vi "generate_list.vi"(9 "Interval":sgl, 10 "End":sgl, 11 "Start":sgl) -> (3 "Array":sgl[](array[numeric]))   [LabVIEW 2020, in "3DPC_SurfacePlot.xctl"]
uses:
  <vilib>/Native 3D Graph/xcontrol/3DPC_SurfacePlot.xctl
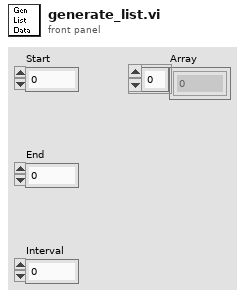
[diagram p1: front panel]
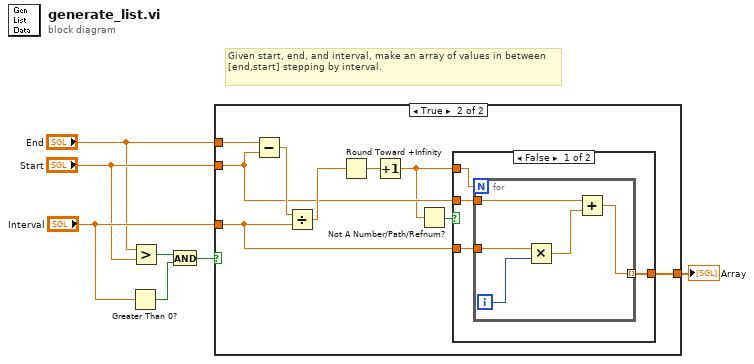
[diagram p0: block diagram]
diagram:
  # "Given start, end, and interval, make an array of values in between [end,start] stepping by interval."
  n1 = Greater Than 0?(x="Interval") -> (x > 0?=w4:bool)
  n2 = Greater?(x="End", y="Start") -> (0:w5:bool)
  n3 = And(x=w5, y=w4) -> (x .and. y?=w3:bool)
  n4 = case shown="True" w3 {
    tunnel: "End" -> [_ w14]
    tunnel: "Interval" -> [_ w12]
    tunnel: "Start" -> [_ w11]
    tunnel: [_ w10] -> w7
    frame False {
    }
    frame True {
      n5 = Subtract(x=w14, y=w11) -> (x-y=w13:sgl)
      n6 = Divide(x=w13, y=w12) -> (x/y=w16:sgl)
      n7 = Round Toward +Infinity(x=w16) -> (ceil(x): smallest int >= x=w15:sgl)
      n8 = Increment(x=w15) -> (x+1=w9:sgl)
      n9 = Not A Number/Path/Refnum?(number/path/refnum=w9) -> (NaN/Path/Refnum?=w8:bool)
      n10 = case shown="False" w8 {
        tunnel: w12 -> [w20 _]
        tunnel: w11 -> [w19 _]
        tunnel: [w18 _] -> w10
        tunnel: w9 -> [w17 _]
        frame False {
          n11 = for {
            N: w17 -> [_]
            tunnel: w20 -> [w25]
            tunnel: w19 -> [w22]
            tunnel: [w21] -> w18 mode=indexing
            i -> [w24]
            n12 = Multiply(x=w25, y=w24) -> (x*y=w23:sgl)
            n13 = Add(x=w22, y=w23) -> (x+y=w21:sgl)
          }
        }
        frame True {
        }
      }
    }
  }
  "Array" <- w7
